vi "Extract_to_spreadsheet.vi"() -> ()   [LabVIEW 2019]
uses:
  SubVIs/TypeDefs/State.ctl
panel:
  in  "Discard":bool
  in  "Accept":bool
  in  "Filename out prefix":string
  out "Harmonic frequencies":dbl[](array[numeric])
  out "Selected harmonic amplitudes":dbl[](array[numeric])
  out "Harmonic amplitudes":dbl[](array[numeric])
  out "Measured frequency":dbl
  out "Signal spectrum":dbl[](graph)
  in  "Harmonics":i32[](array[numeric])
  in  "Calibration factor":dbl
  in  "Lowpass order":i32
  in  "Lowpass cutoff (Hz)":dbl
  out "Progress":u8(slide) scale=0.0..49.0
  out "Current file":string
  in  "Window overlay (s)":dbl
  in  "Sample rate":dbl
  in  "Parse":bool
  in  "stop":bool
  in  "Window length (s)":dbl
  in  "Folder out":path
  in  "Folder in":path
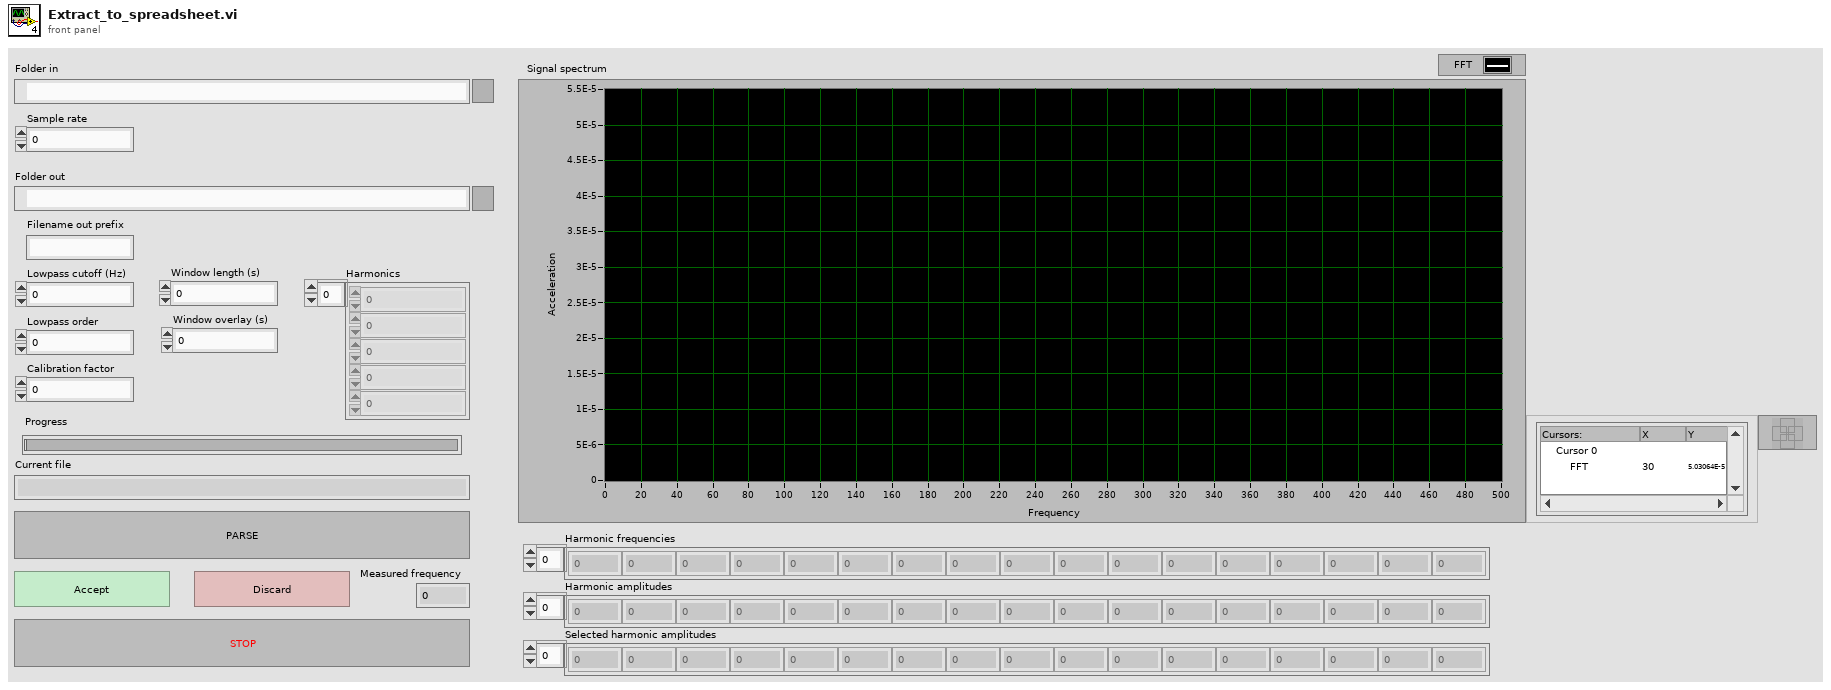
[diagram p1: front panel]
types:
  T1 = typedef "State.ctl" = enum16{"IDLE", "CREATE_HEADER", "SAVE_DATA", "CLOSE"}
  T2 = enum16{"open", "replace", "create", "open or create", "replace or create", "replace or create with confirmation"}
  T3 = enum16{"open", "open or create", "create or replace", "create", "open (read-only)"}
  T4 = cluster{"f":dbl, "x":waveform(dbl), "y":waveform(dbl), "z":waveform(dbl)}
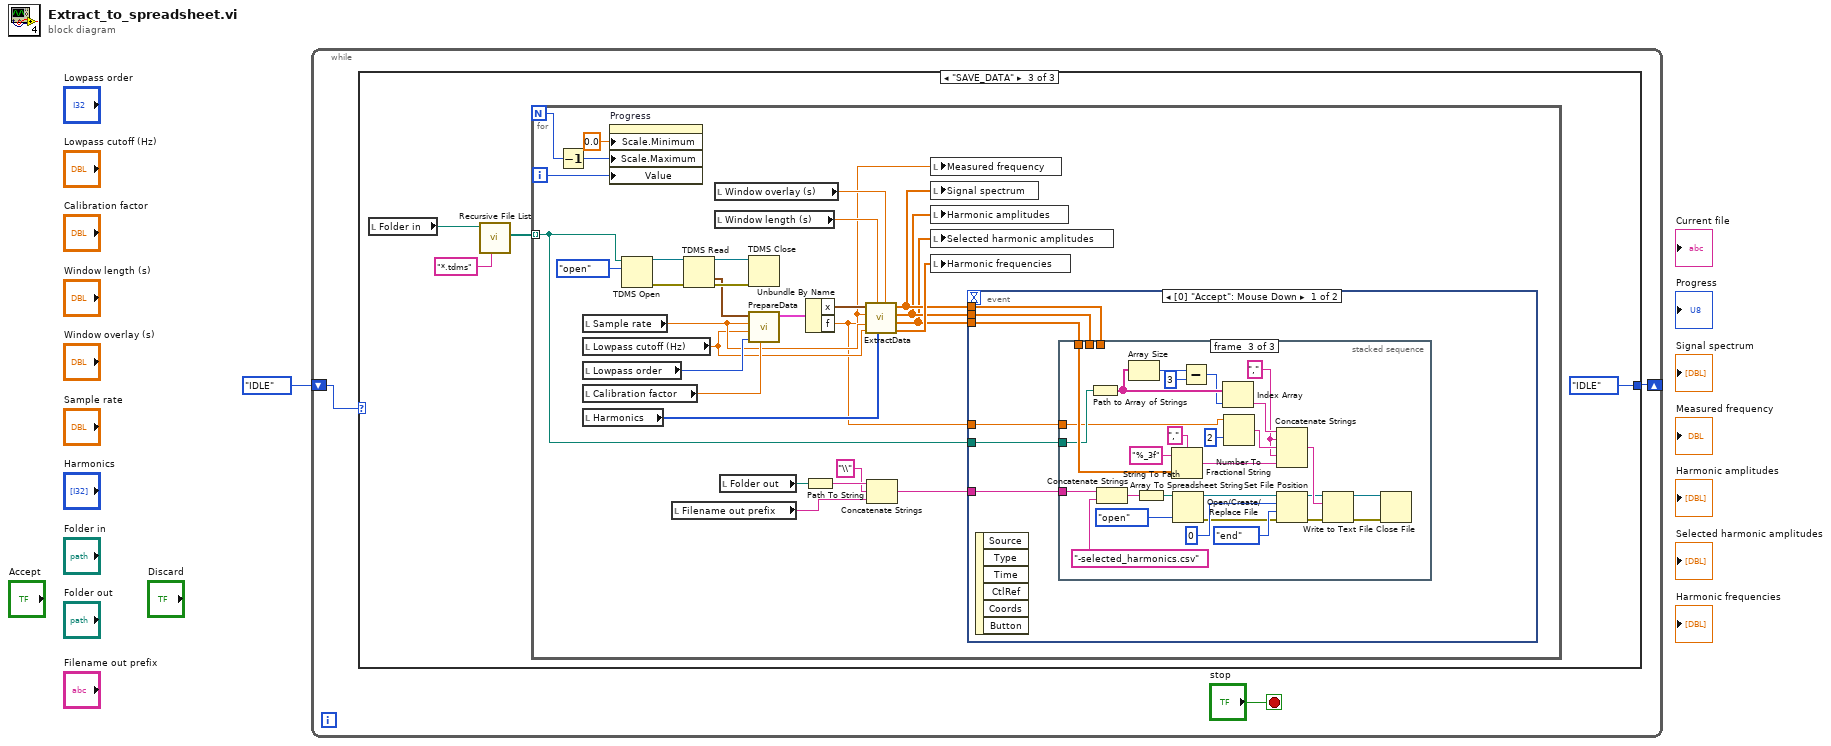
[diagram p0: block diagram]
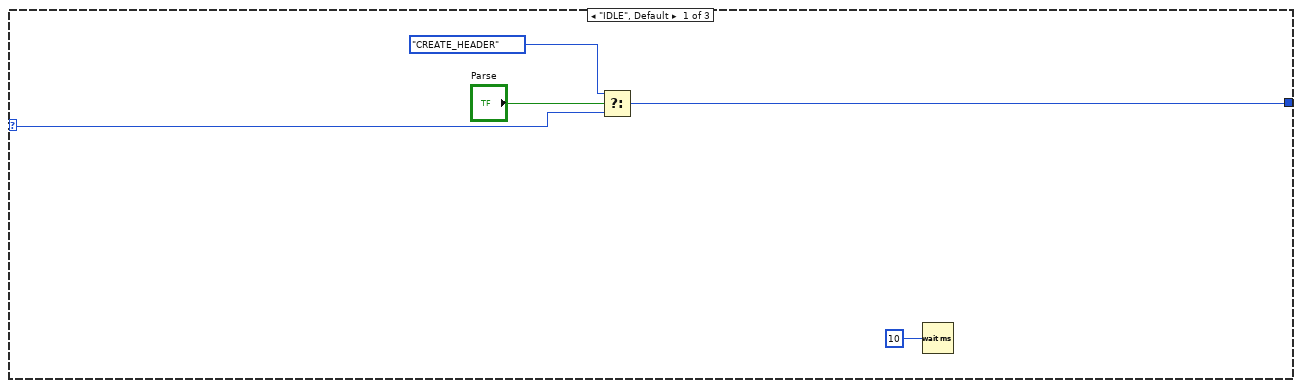
[diagram p2: hidden frame]
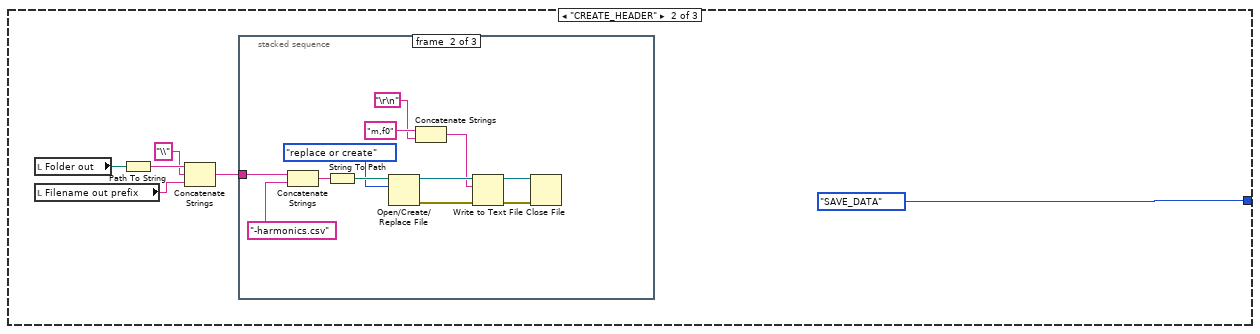
[diagram p3: hidden frame]
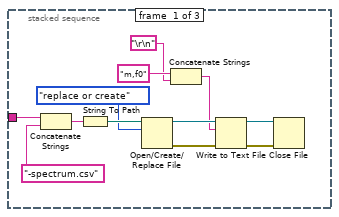
[diagram p4: hidden frame]
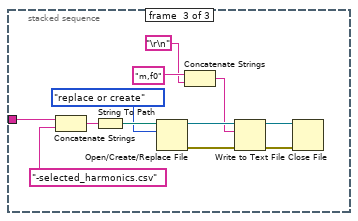
[diagram p5: hidden frame]
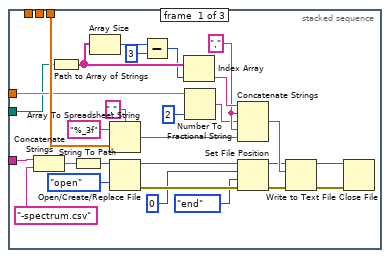
[diagram p6: hidden frame]
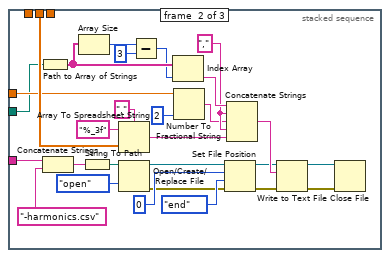
[diagram p7: hidden frame]
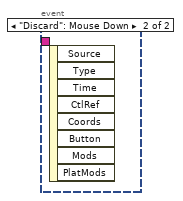
[diagram p8: hidden frame]
diagram:
  n1 = while {
    shift-right: [w4] -> _
    shift-left: State."IDLE" -> [w2]
    stop <- "stop" stop-if-true
    n2 = case shown="\"SAVE_DATA\"" w2 {
      selector: w2 -> [w6 _ _]
      tunnel: [w7 State."SAVE_DATA" State."IDLE"] -> w4
      frame "IDLE", Default {
        n3 = Select(t=State."CREATE_HEADER", s="Parse", f=w6) -> (s? t:f=w7:T1)
        n4 = Wait (ms)(milliseconds to wait=u32 10) -> ()  [unwired: 1 out]
      }
      frame "CREATE_HEADER" {
        n5 = local read "Folder out"() -> (w12:path)
        n6 = local read "Filename out prefix"() -> (w11:string)
        n7 = Path To String(path=w12) -> (string=w14:string)
        n8 = Concatenate Strings(w14, "\\" ("string"), w11) -> (w10:string)
        n9 = stacked-sequence {
          tunnel: w10 -> [w25 w32 w44]
          frame #0 {
            n10 = Concatenate Strings(w25, "-spectrum.csv" ("string")) -> (w26:string)
            n11 = String To Path(string=w26) -> (path=w27:path)
            n12 = Open/Create/Replace File(file path (use dialog)=w27, operation (0:open)=T2."replace or create") -> (refnum out=w22:refnum<file>, error out=w23:errorcluster)  [unwired: 4 in, 1 out]
            n13 = Concatenate Strings("m,f0" ("text"), "\r\n") -> (w17:string)
            n14 = Write to Text File(file (use dialog)=w22, text=w17, error in=w23) -> (refnum out=w20:refnum<file>, error out=w21:errorcluster)  [unwired: 1 in, 1 out]
            n15 = Close File(refnum=w20, error in=w21) -> ()  [unwired: 2 out]
          }
          frame #1 {
            n16 = Concatenate Strings(w32, "-harmonics.csv" ("string")) -> (w38:string)
            n17 = String To Path(string=w38) -> (path=w39:path)
            n18 = Open/Create/Replace File(file path (use dialog)=w39, operation (0:open)=T2."replace or create") -> (refnum out=w36:refnum<file>, error out=w37:errorcluster)  [unwired: 4 in, 1 out]
            n19 = Concatenate Strings("m,f0" ("text"), "\r\n") -> (w28:string)
            n20 = Write to Text File(file (use dialog)=w36, text=w28, error in=w37) -> (refnum out=w34:refnum<file>, error out=w35:errorcluster)  [unwired: 1 in, 1 out]
            n21 = Close File(refnum=w34, error in=w35) -> ()  [unwired: 2 out]
          }
          frame #2 {
            n22 = Concatenate Strings(w44, "-selected_harmonics.csv" ("string")) -> (w50:string)
            n23 = String To Path(string=w50) -> (path=w51:path)
            n24 = Open/Create/Replace File(file path (use dialog)=w51, operation (0:open)=T2."replace or create") -> (refnum out=w48:refnum<file>, error out=w49:errorcluster)  [unwired: 4 in, 1 out]
            n25 = Concatenate Strings("m,f0" ("text"), "\r\n") -> (w41:string)
            n26 = Write to Text File(file (use dialog)=w48, text=w41, error in=w49) -> (refnum out=w46:refnum<file>, error out=w47:errorcluster)  [unwired: 1 in, 1 out]
            n27 = Close File(refnum=w46, error in=w47) -> ()  [unwired: 2 out]
          }
        }
      }
      frame "SAVE_DATA" {
        n28 = local read "Folder in"() -> (w53:path)
        n29 = call <vilib>:"Recursive File List.vi"("pattern"="*.tdms", "Folder Path"=w53) -> ("All Files in Dir"=w54:path[])  [unwired: 5 in, 4 out]
        n30 = for {
          N -> [w79]
          tunnel: w54 -> [w57] mode=indexing
          i -> [w78]
          n31 = Decrement(x=w79) -> (x-1=w77:i32)
          n32 = local read "Sample rate"() -> (w72:dbl)
          n33 = local read "Lowpass cutoff (Hz)"() -> (w71:dbl)
          n34 = local read "Lowpass order"() -> (w73:i32)
          n35 = local read "Calibration factor"() -> (w74:dbl)
          n36 = local read "Harmonics"() -> (w70:i32[])
          n37 = property on="Progress" class="Slide (strict)"("Scale.Minimum"=0.0 ("Scale.Range:Minimum"), "Scale.Maximum"=w77, "Value"=w78) -> ()  [unwired: 2 in, 2 out]
          n38 = TDMS Open(10:T3."open" ("operation (0:open)"), 11:w57) -> (0:w83:errorcluster, 3:w84:refnum<k34>)  [unwired: 5 in]
          n39 = local read "Filename out prefix"() -> (w63:string)
          n40 = TDMS Read(0:w84, 11:w83) -> (4:w82:refnum<k34>, 10:w76:waveform(dbl)[], 15:w81:errorcluster)  [unwired: 6 in, 3 out]
          n41 = local read "Window overlay (s)"() -> (w68:dbl)
          n42 = local read "Window length (s)"() -> (w69:dbl)
          n43 = local read "Folder out"() -> (w65:path)
          n44 = TDMS Close(8:w81, 11:w82) -> ()  [unwired: 2 out]
          n45 = call "PrepareData.vi"("Calibration factor"=w74, "Lowpass order"=w73, "Lowpass cutoff"=w71, "Sampling frequecy"=w72, "3 axis + tacho"=w76) -> ("3 axis + frequency"=w75:T4)  [unwired: 6 in]
          n46 = Path To String(path=w65) -> (string=w64:string)
          n47 = Unbundle By Name(w75) -> ("x"=w67:waveform(dbl), "f"=w56:dbl)
          n48 = call "ExtractData.vi"("Window overlay (s)"=w68, "Harmonics"=w70, "Window length (s)"=w69, "Frequency limit"=w71, "Sampling frequency"=w72, "Frequency (f0)"=w56, "Signal in"=w67) -> ("Harmonic frequencies"=w66:dbl[], "Selected harmonics"=w58:dbl[], "Harmonics"=w59:dbl[], "Spectrum"=w60:dbl[])  [unwired: 1 in]
          n49 = Concatenate Strings(w64, "\\" ("string"), w63) -> (w61:string)
          n50 = local write "Measured frequency"(w56) -> ()
          n51 = local write "Signal spectrum"(w60) -> ()
          n52 = local write "Harmonic amplitudes"(w59) -> ()
          n53 = local write "Selected harmonic amplitudes"(w58) -> ()
          n54 = local write "Harmonic frequencies"(w66) -> ()
          n55 = event shown="[0] \"Accept\": Mouse Down" {
            selector: _ -> [_ _]
            dyn-events: _ -> [_ _]
            timeout: _ -> [_ _]
            tunnel: w61 -> [w91 _]
            tunnel: w60 -> [w90 _]
            tunnel: w59 -> [w89 _]
            tunnel: w58 -> [w88 _]
            tunnel: w57 -> [w87 _]
            tunnel: w56 -> [w86 _]
            event "Accept": Mouse Down {
              n56 = event-data() -> ()  [unwired: 1 in, 6 out]
              n57 = stacked-sequence {
                tunnel: w91 -> [w117 w140 w168]
                tunnel: w90 -> [w114 _ _]
                tunnel: w89 -> [_ w139 _]
                tunnel: w88 -> [_ _ w167]
                tunnel: w87 -> [w104 w132 w166]
                tunnel: w86 -> [w105 w133 w160]
                frame #0 {
                  w103 = "," ("string")
                  n58 = Concatenate Strings(w117, "-spectrum.csv" ("string")) -> (w118:string)
                  n59 = Path to Array of Strings(0:w104) -> (2:w109:string[])  [unwired: 1 out]
                  n60 = String To Path(string=w118) -> (path=w119:path)
                  n61 = Array Size(array=w109) -> (size(s)=w99:i32)
                  n62 = Array To Spreadsheet String(delimiter (Tab)=",", array=w114, 3:"%_3f" ("format string")) -> (spreadsheet string=w101:string)
                  n63 = Open/Create/Replace File(file path (use dialog)=w119, operation (0:open)=T2."open") -> (refnum out=w97:refnum<file>, error out=w95:errorcluster)  [unwired: 4 in, 1 out]
                  n64 = Subtract(x=w99, y=3) -> (x-y=w107:i32)
                  n65 = Index Array(array=w109, index=w107) -> (element=w106:string)
                  n66 = Number To Fractional String(number=w105, precision (6)=i16 2) -> (F-format string=w102:string)  [unwired: 2 in]
                  n67 = Concatenate Strings(w106, w103, w102, w103, w101) -> (w100:string)
                  n68 = Set File Position(offset (in bytes) (0)=i64 0, refnum=w97, from (0:start)=enum16{"start", "end", "current"}."end", error in=w95) -> (refnum out=w96:refnum<file>, error out=w94:errorcluster)
                  n69 = Write to Text File(file (use dialog)=w96, text=w100, error in=w94) -> (refnum out=w111:refnum<file>, error out=w112:errorcluster)  [unwired: 1 in, 1 out]
                  n70 = Close File(refnum=w111, error in=w112) -> ()  [unwired: 2 out]
                }
                frame #1 {
                  w131 = "," ("string")
                  n71 = Path to Array of Strings(0:w132) -> (2:w137:string[])  [unwired: 1 out]
                  n72 = Concatenate Strings(w140, "-harmonics.csv" ("string")) -> (w146:string)
                  n73 = Array Size(array=w137) -> (size(s)=w127:i32)
                  n74 = String To Path(string=w146) -> (path=w147:path)
                  n75 = Array To Spreadsheet String(delimiter (Tab)=",", array=w139, 3:"%_3f" ("format string")) -> (spreadsheet string=w128:string)
                  n76 = Open/Create/Replace File(file path (use dialog)=w147, operation (0:open)=T2."open") -> (refnum out=w122:refnum<file>, error out=w123:errorcluster)  [unwired: 4 in, 1 out]
                  n77 = Subtract(x=w127, y=3) -> (x-y=w135:i32)
                  n78 = Index Array(array=w137, index=w135) -> (element=w134:string)
                  n79 = Number To Fractional String(number=w133, precision (6)=i16 2) -> (F-format string=w130:string)  [unwired: 2 in]
                  n80 = Set File Position(offset (in bytes) (0)=i64 0, refnum=w122, from (0:start)=enum16{"start", "end", "current"}."end", error in=w123) -> (refnum out=w121:refnum<file>, error out=w120:errorcluster)
                  n81 = Concatenate Strings(w134, w131, w130, w131, w128) -> (w129:string)
                  n82 = Write to Text File(file (use dialog)=w121, text=w129, error in=w120) -> (refnum out=w141:refnum<file>, error out=w142:errorcluster)  [unwired: 1 in, 1 out]
                  n83 = Close File(refnum=w141, error in=w142) -> ()  [unwired: 2 out]
                }
                frame #2 {
                  w156 = "," ("string")
                  n84 = Path to Array of Strings(0:w166) -> (2:w165:string[])  [unwired: 1 out]
                  n85 = Concatenate Strings(w168, "-selected_harmonics.csv" ("string")) -> (w174:string)
                  n86 = Array Size(array=w165) -> (size(s)=w164:i32)
                  n87 = String To Path(string=w174) -> (path=w175:path)
                  n88 = Array To Spreadsheet String(delimiter (Tab)=",", array=w167, 3:"%_3f" ("format string")) -> (spreadsheet string=w159:string)
                  n89 = Open/Create/Replace File(file path (use dialog)=w175, operation (0:open)=T2."open") -> (refnum out=w152:refnum<file>, error out=w151:errorcluster)  [unwired: 4 in, 1 out]
                  n90 = Subtract(x=w164, y=3) -> (x-y=w162:i32)
                  n91 = Index Array(array=w165, index=w162) -> (element=w157:string)
                  n92 = Number To Fractional String(number=w160, precision (6)=i16 2) -> (F-format string=w158:string)  [unwired: 2 in]
                  n93 = Concatenate Strings(w157, w156, w158, w156, w159) -> (w155:string)
                  n94 = Set File Position(offset (in bytes) (0)=i64 0, refnum=w152, from (0:start)=enum16{"start", "end", "current"}."end", error in=w151) -> (refnum out=w149:refnum<file>, error out=w148:errorcluster)
                  n95 = Write to Text File(file (use dialog)=w149, text=w155, error in=w148) -> (refnum out=w169:refnum<file>, error out=w170:errorcluster)  [unwired: 1 in, 1 out]
                  n96 = Close File(refnum=w169, error in=w170) -> ()  [unwired: 2 out]
                }
              }
            }
            event "Discard": Mouse Down {
              n97 = event-data() -> ()  [unwired: 1 in, 8 out]
            }
          }
        }
      }
    }
  }
